vi "Set Matrix - stdin.vi"(8 "error in":errorcluster, 9 "value":dbl[][](array[numeric]), 10 "variable name":string, 11 "GOLPI ref. in":T1={"pipe handle"={"lv_proc.dll file path"=path "", "process instance handle"=[]}, "fast read timeout [ms]"=500, "fast read settle time [ms]"=10, "fast read to multiple [ms]"=1, "max elements per input line"=100}) -> (0 "error out":errorcluster, 3 "GOLPI ref. out":T1={"pipe handle"={"lv_proc.dll file path"=path "", "process instance handle"=[]}, "fast read timeout [ms]"=500, "fast read settle time [ms]"=10, "fast read to multiple [ms]"=1, "max elements per input line"=100})   [LabVIEW 2013, in "GOLPI library.lvlib"]
uses:
  GOLPI library.lvlib
  Type Definitions/GOLPI reference Type Def.ctl
  LV Process.lvlibp/Pipe Handle.ctl
  LV Process.lvlibp
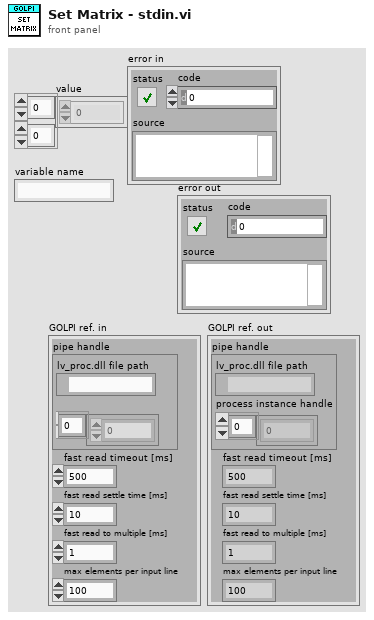
[diagram p1: front panel]
types:
  T1 = typedef "GOLPI library.lvlib/GOLPI reference Type Def.ctl" = cluster{"pipe handle":T2, "fast read timeout [ms]":u32, "fast read settle time [ms]":u32, "fast read to multiple [ms]":u32, "max elements per input line":u32}
  T2 = typedef "LV Process.lvlibp/Pipe Handle.ctl" = cluster{"lv_proc.dll file path":path, "process instance handle":u32[]}
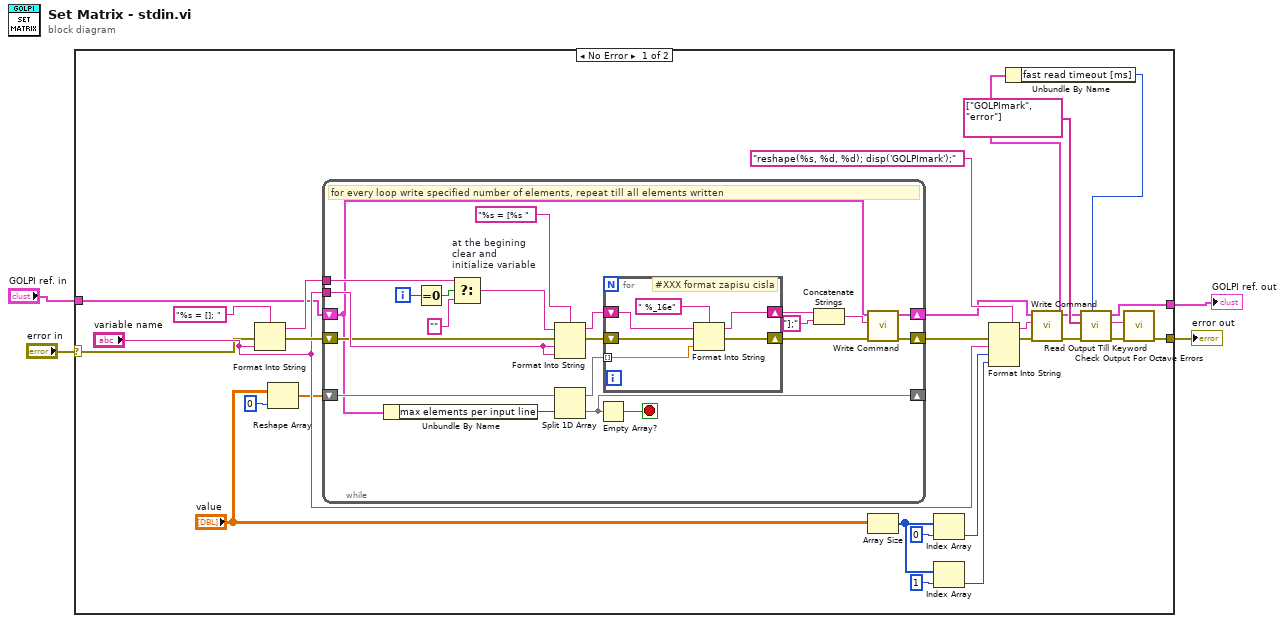
[diagram p0: block diagram]
diagram:
  n1 = case shown="No Error" "error in" {
    selector: "error in" -> [w9 w61]
    tunnel: [w10 w61] -> w4
    tunnel: "GOLPI ref. in" -> [w8 w60]
    tunnel: [w7 w60] -> w2
    frame No Error {
      n2 = Format Into String(format string="%s = []; ", error in=w9, "variable name") -> (resulting string=w18:string, error out=w30:errorcluster)  [unwired: 1 in]
      n3 = Reshape Array("value", 0 ("dimension size")) -> (w20:dbl[])
      n4 = while {
        shift-right: [w52] -> _
        shift-left: w20 -> [w53]
        tunnel: "variable name" -> [w45]
        shift-right: [w41] -> w31
        shift-left: w30 -> [w44]
        shift-right: [w40] -> w15
        shift-left: w8 -> [w32]
        tunnel: w18 -> [w36]
        i -> [w38]
        stop <- w51 stop-if-true
        # "for every loop write specified number of elements, repeat till all elements written"
        n5 = Unbundle By Name(w32) -> ("max elements per input line"=w33:u32)
        n6 = Equal To 0?(x=w38) -> (x = 0?=w37:bool)
        n7 = Select "at the begining\nclear and\ninitialize variable"(t=w36, s=w37, f="") -> (s? t:f=w35:string)
        n8 = Format Into String(format string="%s = [%s ", initial string=w35, error in=w44, w45, w45) -> (resulting string=w48:string, error out=w43:errorcluster)
        n9 = Split 1D Array(array=w53, index=w33) -> (first subarray=w49:dbl[], second subarray=w52:dbl[])
        n10 = Empty Array?(array=w52) -> (empty?=w51:bool)
        n11 = for {
          tunnel: w49 -> [w59] mode=indexing
          shift-right: [w57] -> w47
          shift-left: w48 -> [w56]
          shift-right: [w54] -> w42
          shift-left: w43 -> [w55]
          # "#XXX format zapisu cisla"
          n12 = Format Into String(format string=" %_16e", initial string=w56, error in=w55, w59) -> (resulting string=w57:string, error out=w54:errorcluster)
        }
        n13 = Concatenate Strings(w47, "];" ("string")) -> (w39:string)
        n14 = call "Write Command.vi"("error in"=w42, "command"=w39, "GOLPI ref. in"=w32) -> ("error out"=w41:errorcluster, "GOLPI ref. out"=w40:T1)  [unwired: 7 in]
      }
      n15 = Array Size(array="value") -> (size(s)=w25:i32[])
      n16 = Index Array(array=w25, index=0) -> (element=w28:i32)
      n17 = Index Array(array=w25, index=1) -> (element=w29:i32)
      n18 = Format Into String(format string="reshape(%s, %d, %d); disp('GOLPImark');", error in=w31, "variable name", w28, w29) -> (resulting string=w17:string, error out=w16:errorcluster)  [unwired: 1 in]
      n19 = call "Write Command.vi"("error in"=w16, "command"=w17, "GOLPI ref. in"=w15) -> ("error out"=w11:errorcluster, "GOLPI ref. out"=w6:T1)  [unwired: 7 in]
      n20 = Unbundle By Name(w6) -> ("fast read timeout [ms]"=w5:u32)
      n21 = call "Read Output Till Keyword.vi"("timeout [ms]"=w5, "error in"=w11, "keywords"=string[] ["GOLPImark", "error"], "GOLPI ref. in"=w6) -> ("error out"=w14:errorcluster, "read buffer"=w12:string, "GOLPI ref. out"=w7:T1)  [unwired: 4 in, 1 out]
      n22 = call "Check Output For Octave Errors.vi"("error in"=w14, "read buffer"=w12) -> ("error out"=w10:errorcluster)  [unwired: 9 in]
    }
    frame Error {
    }
  }
  "error out" <- w4
  "GOLPI ref. out" <- w2
